vi "Choreo_EventMarker_OffsetBy.vi"(9 "TimestampOffset":dbl, 11 "EventMarker":T1) -> (3 "offsetEventMarker":T1)   [LabVIEW 2019, in "ChoreoLib.lvlib"]
doc: "Create a list of event markers from json string\n\nInputs:\n - JSONString - string - String potentially containing an event marker\n\nOutputs:\n - EventMarkers - array of cluster - The event markers defined by the given json object\n - Exists - boolean- TRUE if any event markers were found in the JSON string.\n\nNotes:\n--------\nCurrently the only type of commands that can be issued are Boolean commands. The value is forced to TRUE when the command is issued.\n\nThe following table lists the actions performed for different types of commands:\n - Unknown - nothing - not supported.\n - Wait - nothing - not supported\n - Named - Issue boolean command with TRUE value using the \"name\" as the command name.\n - Path - nothing - not supported\n - Sequential, Parallel, Race, Deadline - Issue boolean command with TRUE value for each of the commands contained in the \"commands\" array. The value for \"name\" is used as the command name."
uses:
  ChoreoLib.lvlib
  TypeDef/ChoreoEventMarker.ctl
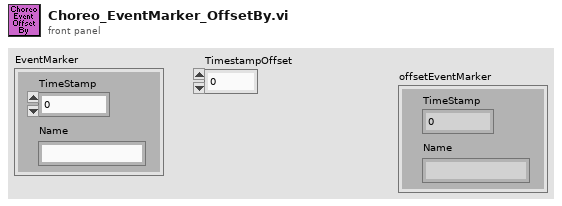
[diagram p1: front panel]
types:
  T1 = typedef "ChoreoLib.lvlib/ChoreoEventMarker.ctl" = cluster{"TimeStamp":dbl, "Name":string}
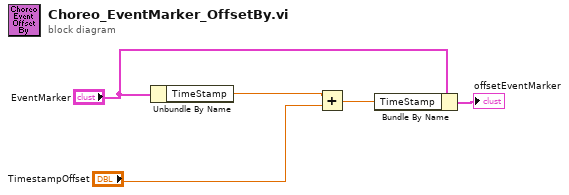
[diagram p0: block diagram]
diagram:
  n1 = Unbundle By Name("EventMarker") -> ("TimeStamp"=w3:dbl)
  n2 = Add(x=w3, y="TimestampOffset") -> (x+y=w2:dbl)
  n3 = Bundle By Name(cluster="EventMarker", "TimeStamp"=w2) -> (→"offsetEventMarker":T1)
